vi "sub_query_donCheck.vi"(0 "error in (no error)":errorcluster) -> (3 "error out":errorcluster)   [LabVIEW 2019]
uses:
  _ctrl/init-r-stop.ctl
  Durability/common/Global 1.vi
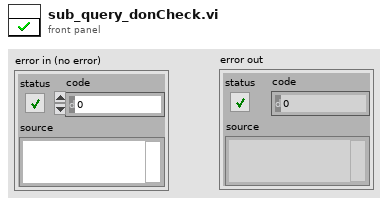
[diagram p1: front panel]
types:
  T1 = typedef "init-r-stop.ctl" = enum16{"ini", "read", "stop"}
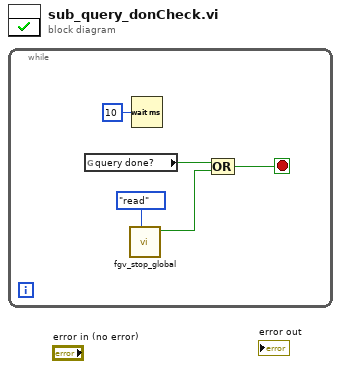
[diagram p0: block diagram]
diagram:
  n1 = while {
    stop <- w3 stop-if-true
    n2 = global read "Global 1.vi" "query done?"() -> (w4:bool)
    n3 = call "fgv_stop_global.vi"("cmd"=init-r-stop."read") -> ("stop"=w1:bool)  [unwired: 10 in]
    n4 = Wait (ms)(milliseconds to wait=u32 10) -> ()  [unwired: 1 out]
    n5 = Compound Arithmetic op=OR(w4, w1) -> (w3:bool)
  }
